vi "GET_ignition_status.vi"(8 "API Key":string="cheia04042025tema2restfulapi") -> (0 "body":string, 1 "headers":string, 2 "ign_stat":cluster{"ign_stat":string})   [LabVIEW 2024]
uses:
  <vilib>/httpClient/LabVIEWHTTPClient.lvlib
panel:
  out "error out":errorcluster
  out "error out get":errorcluster
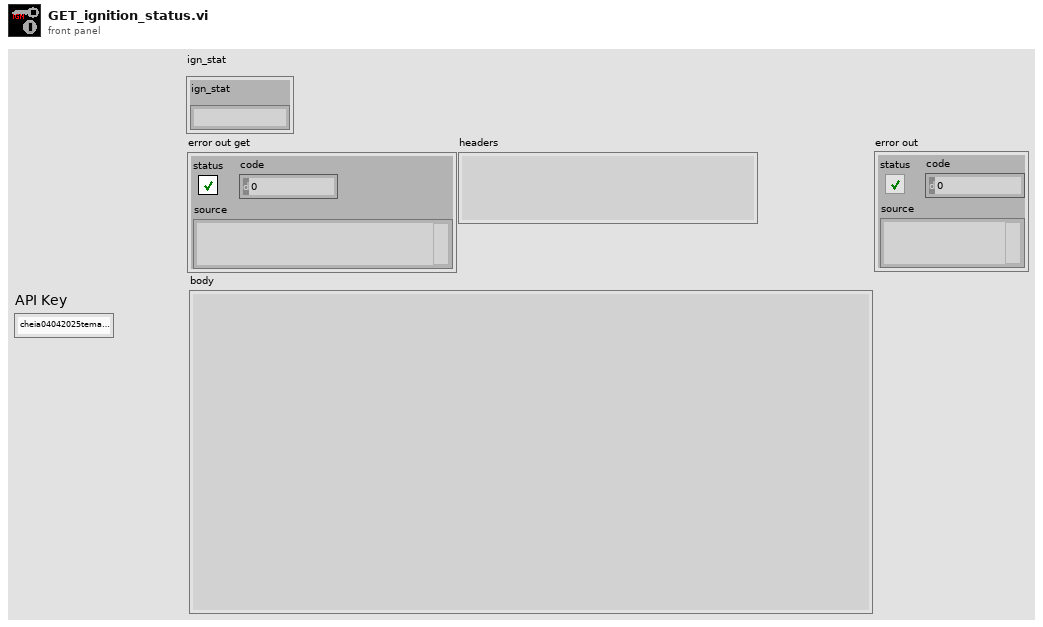
[diagram p1: front panel]
types:
  T1 = typedef "LabVIEWHTTPClient.lvlib/ClientHandle.ctl" = refnum<k1>
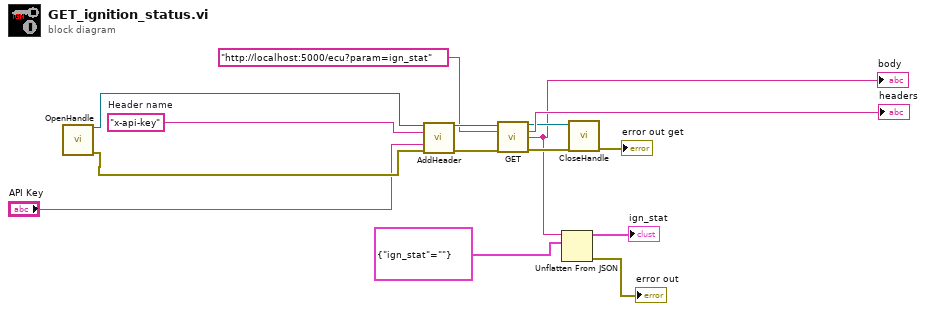
[diagram p0: block diagram]
diagram:
  w7 = "x-api-key"  # Header name
  n1 = call <vilib>:"OpenHandle.vi"() -> ("client handle out"=w8:T1, "error out"=w9:errorcluster)  [unwired: 14 in]
  n2 = call <vilib>:"AddHeader.vi"("client handle"=w8, "header"=w7, "value"="API Key", "error in (no error)"=w9) -> ("client handle out"=w11:T1, "error out"=w10:errorcluster)  [unwired: 10 in]
  n3 = call <vilib>:"GET.vi"("client handle"=w11, "url"="http://localhost:5000/ecu?param=ign_stat", "error in (no error)"=w10) -> ("client handle out"=w13:T1, "headers"=→"headers":string, "body"=w3:string, "error out"=w12:errorcluster)  [unwired: 9 in]
  "body" <- w3
  n4 = Unflatten From JSON(JSON string=w3, type and defaults=cluster{"ign_stat":string} {"ign_stat"=""}) -> (value=→"ign_stat":cluster{"ign_stat":string}, error out=→"error out":errorcluster)  [unwired: 5 in]
  n5 = call <vilib>:"CloseHandle.vi"("client handle"=w13, "error in (no error)"=w12) -> ("error out"=→"error out get":errorcluster)  [unwired: 13 in]
